vi "ReadValByRefArrU16.vi"(0 "Refs":refnum<vi>[](array[refnum]), 2 "Type In":u16, 5 "Ref_Idx":i32, 11 "error in":errorcluster caption="entrée d'erreur") -> (4 "Valeur":u16, 15 "error out":errorcluster caption="sortie d'erreur")   [LabVIEW 2019]
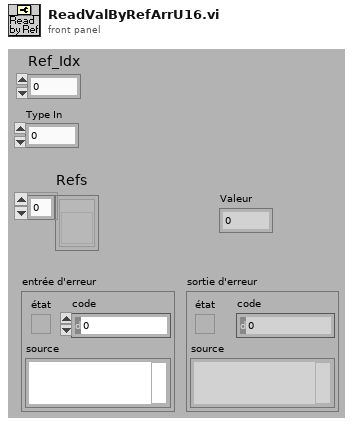
[diagram p1: front panel]
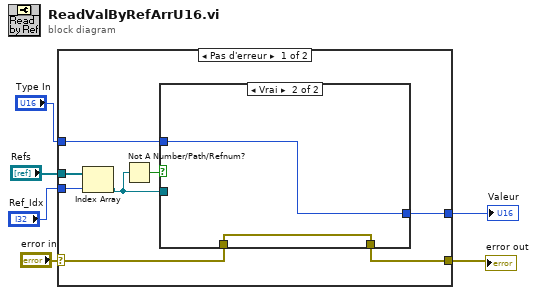
[diagram p0: block diagram]
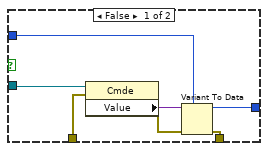
[diagram p2: hidden frame]
diagram:
  n1 = case shown="Pas d'erreur" "error in" {
    selector: "error in" -> [w12 w24]
    tunnel: [w13 _] -> w6
    tunnel: [w11 w24] -> w4
    tunnel: "Type In" -> [w10 _]
    tunnel: "Refs" -> [w9 _]
    tunnel: "Ref_Idx" -> [w8 _]
    frame No Error {
      n2 = Index Array(array=w9, index=w8) -> (element=w7:refnum<vi>)
      n3 = Not A Number/Path/Refnum?(number/path/refnum=w7) -> (NaN/Path/Refnum?=w14:bool)
      n4 = case shown="Vrai" w14 {
        tunnel: w7 -> [w21 _]
        tunnel: [w19 w22] -> w13
        tunnel: w12 -> [w16 w23]
        tunnel: [w18 w23] -> w11
        tunnel: w10 -> [w17 w22]
        frame False {
          n5 = property class="Cmde"(reference=w21, error in=w16) -> (error out=w15:errorcluster, "Value"=w20:variant)  [unwired: 1 out]
          n6 = Variant To Data(error in=w15, type=w17, Variant=w20) -> (data=w19:u16, error out=w18:errorcluster)
        }
        frame True {
        }
      }
    }
    frame Error {
    }
  }
  "Valeur" <- w6
  "error out" <- w4
